vi "WPI_SerialPortFlush.vi"(8 "error in (no error)":errorcluster, 11 "SerialPortRef":T1) -> (0 "error out":errorcluster, 3 "SerialPortRef":T1)   [LabVIEW 2017]
doc: "Flushes and discards contents of the output buffer of the serial device you specify by writing all the buffered data to the device.\n\nThis software is licensed. Open the labview\\readme\\WPI Robotics Library Open Source License.txt file for more information."
uses:
  <vilib>/Rock Robotics/WPI/SerialPort/WPI_SerialPortRef.ctl
  <vilib>/Instr/_visa.llb/VISA Flush IO Buffer Mask.ctl
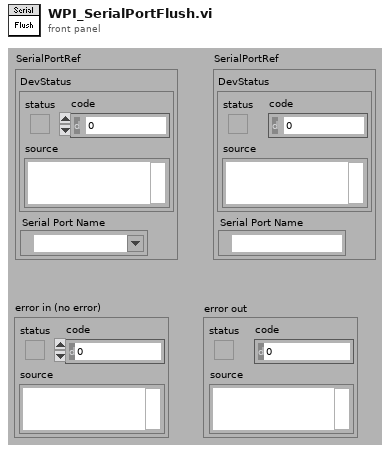
[diagram p1: front panel]
types:
  T1 = typedef "WPI_SerialPortRef.ctl" = cluster{"DevStatus":errorcluster, "Serial Port Name":refnum<visa-resource-name>}
  T2 = typedef "VISA Flush IO Buffer Mask.ctl" = u16
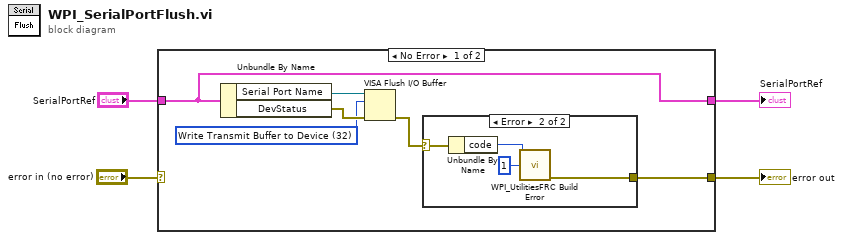
[diagram p0: block diagram]
diagram:
  n1 = case shown="No Error" "error in (no error)" {
    selector: "error in (no error)" -> [_ w17]
    tunnel: "SerialPortRef" -> [w5 w16]
    tunnel: [w5 w16] -> w3
    tunnel: [w6 w17] -> w1
    frame No Error {
      w8 = T2 32 items=["Flush Receive Buffer"=16, "Write Transmit Buffer to Device"=32, "Flush Receive Buffer (No I/O)"=64, "Flush Transmit Buffer"=128] ("Mask")
      n2 = Unbundle By Name(w5) -> ("Serial Port Name"=w10:refnum<visa-resource-name>, "DevStatus"=w9:errorcluster)
      n3 = VISA Flush I/O Buffer(VISA resource name=w10, mask (16)=w8, error in (no error)=w9) -> (error out=w7:errorcluster)  [unwired: 1 out]
      n4 = case shown="Error" w7 {
        selector: w7 -> [w11 w13]
        tunnel: [w11 w12] -> w6
        frame No Error {
        }
        frame Error {
          n5 = Unbundle By Name(w13) -> ("code"=w15:i32)
          n6 = call <vilib>:"WPI_UtilitiesFRC Build Error.vi"("error code"=w15, "chain levels to remove (1)"=1) -> ("error out"=w12:errorcluster)  [unwired: 3 in, 10 out]
        }
      }
    }
    frame Error {
    }
  }
  "error out" <- w1
  "SerialPortRef" <- w3
